vi "Message Window GUI.vi"() -> ()   [LabVIEW 2022 SP3, in "Generic Utilities.lvclass"]
uses:
  Generic Utilities.lvclass
panel:
  in  "Message":string="\nPlease Wait...\n\nProcessing!"
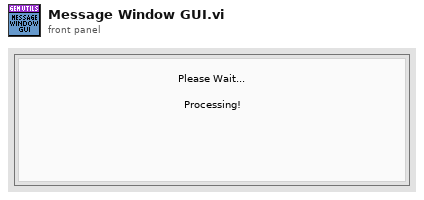
[diagram p1: front panel]
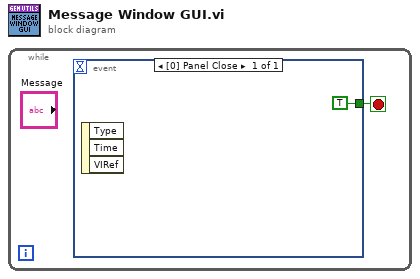
[diagram p0: block diagram]
diagram:
  n1 = while {
    stop <- w1 stop-if-true
    n2 = event shown="[0] Panel Close" {
      selector: _ -> [_]
      dyn-events: _ -> [_]
      timeout: _ -> [_]
      tunnel: [TRUE] -> w1
      event Panel Close {
        n3 = event-data() -> ()  [unwired: 1 in, 3 out]
      }
    }
  }
